vi "Drawing a Filled Circle.vi"(10 "number of points":i32=180, 11 "circle":cluster{"x0":dbl, "y0":dbl, "r":dbl}) -> (3 "circle graph":cluster{"x":dbl[], "y":dbl[]})   [LabVIEW 2023]
doc: "Convert a circle x0, y0, and r values into arrays of X and Y values that can be used to draw a filled circle in an XY Graph."
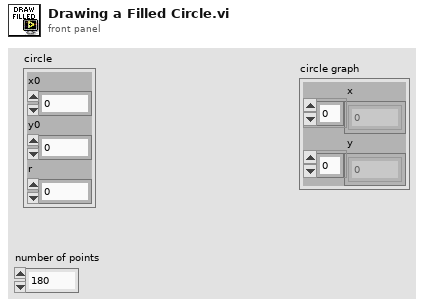
[diagram p1: front panel]
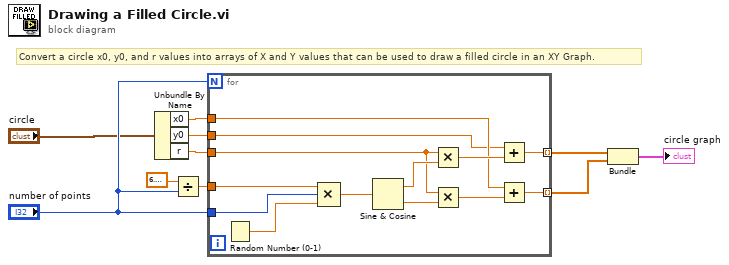
[diagram p0: block diagram]
diagram:
  # "Convert a circle x0, y0, and r values into arrays of X and Y values that can be used to draw a filled circle in an XY Graph."
  n1 = Unbundle By Name("circle") -> ("x0"=w3:dbl, "y0"=w2:dbl, "r"=w1:dbl)
  n2 = Divide(x=6.283185307179586, y="number of points") -> (x/y=w9:dbl)
  n3 = for {
    N: "number of points" -> [_]
    tunnel: w9 -> [w14]
    tunnel: w3 -> [w20]
    tunnel: [w18] -> w8 mode=indexing
    tunnel: [w17] -> w7 mode=indexing
    tunnel: "number of points" -> [w13]
    tunnel: w2 -> [w16]
    tunnel: w1 -> [w15]
    n4 = Random Number (0-1)() -> (number: 0 to 1=w12:dbl)
    n5 = Compound Arithmetic op=MULTIPLY(w14, w13, w12) -> (w11:dbl)
    n6 = Sine & Cosine(0:w11) -> (1:w23:dbl, 2:w22:dbl)
    n7 = Multiply(x=w15, y=w23) -> (x*y=w21:dbl)
    n8 = Multiply(x=w15, y=w22) -> (x*y=w19:dbl)
    n9 = Add(x=w16, y=w21) -> (x+y=w18:dbl)
    n10 = Add(x=w20, y=w19) -> (x+y=w17:dbl)
  }
  n11 = Bundle(w8, w7) -> (→"circle graph":cluster{dbl[], dbl[]})  [unwired: 1 in]
